vi "Insert Add States to Queue.vi"(8 "error in (no error)":errorcluster, 9 "Mouse Position":T1, 10 "Variant in":path, 11 "?":refnum<vi>) -> (0 "error out":errorcluster)   [LabVIEW 2020]
doc: "Inserts the object specified by name in the Quick Drop dialog box on the selected wire(s) on the diagram. If [Shift] is also pressed, and multiple wires were selected, a single instance of the object is inserted on those wires.\n\nDefault Shortcut - [I]"
uses:
  <vilib>/Utility/miscctls.llb/LVPositionTypeDef.ctl
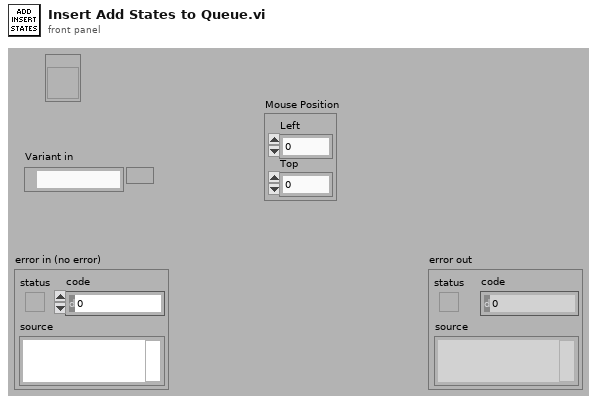
[diagram p1: front panel]
types:
  T1 = typedef "LVPositionTypeDef.ctl" = cluster{"Left":i32, "Top":i32}
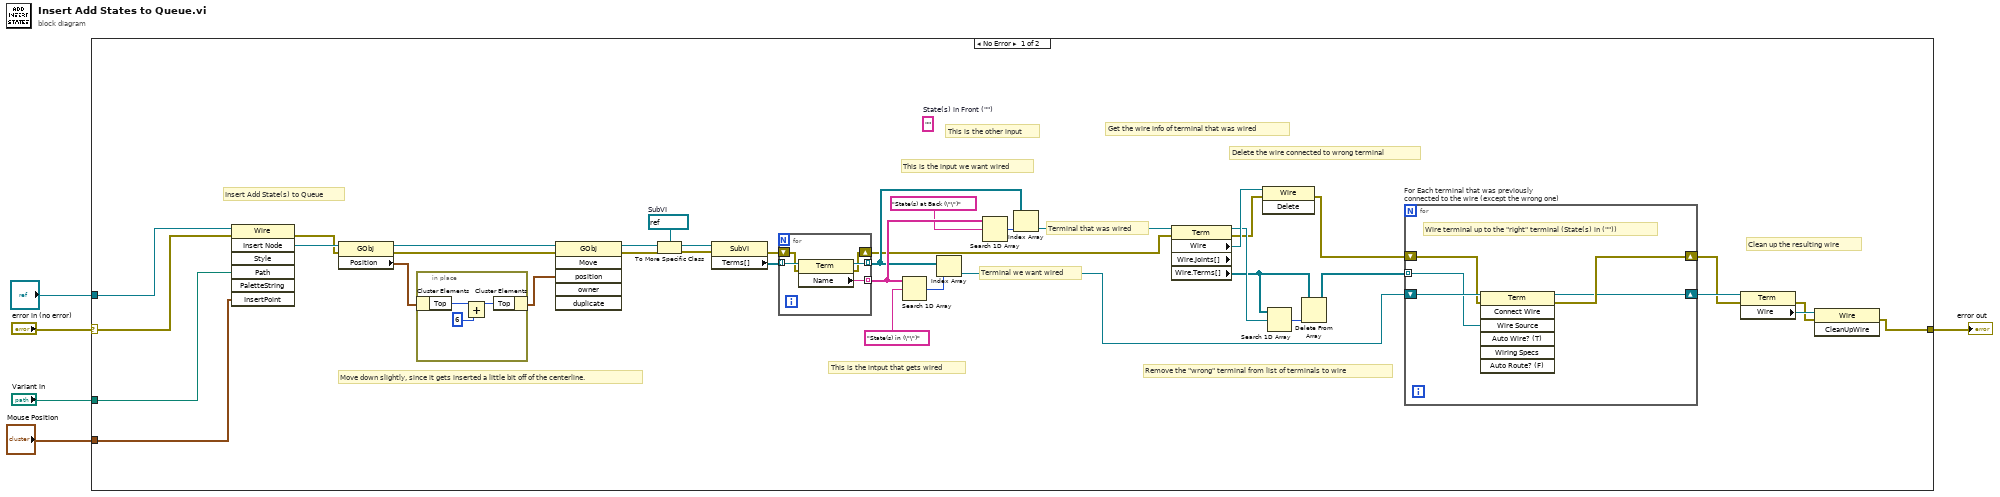
[diagram p0: block diagram]
diagram:
  n1 = case shown="No Error" "error in (no error)" {
    selector: "error in (no error)" -> [w42 w57]
    tunnel: [w43 w57] -> w4
    tunnel: "Variant in" -> [w41 _]
    tunnel: "?" -> [w40 _]
    tunnel: "Mouse Position" -> [w39 _]
    frame No Error {
      w38 = refnum<vi> refnum  # SubVI
      (unwired) ""  # State(s) in Front ("")
      # "Clean up the resulting wire"
      # "Remove the \"wrong\" terminal from list of terminals to wire"
      # "Delete the wire connected to wrong terminal"
      # "Get the wire info of terminal that was wired"
      # "This is the other input"
      # "This is the input we want wired"
      # "This is the intput that gets wired"
      # "Insert Add State(s) to Queue"
      # "Move down slightly, since it gets inserted a little bit off of the centerline."
      # "Terminal that was wired"
      # "Terminal we want wired"
      n2 = invoke class="Wire" method="Insert Node"(reference=w40, error in=w42, "Path"=w41, "InsertPoint"=w39) -> (error out=w11:errorcluster, "Insert Node"=w12:refnum<vi>)  [unwired: 3 in, 5 out]
      n3 = property class="GObj"(reference=w12, error in=w11) -> (reference out=w10:refnum<vi>, error out=w7:errorcluster, "Position"=w13:T1)
      n4 = in-place {
        n5 = in-place-cluster #1(w13) -> ("Top"=w46:i32)
        n6 = Add(x=w46, y=6) -> (x+y=w44:i32)
        n7 = in-place-cluster #1("Top"=w44) -> (w8:T1)
      }
      n8 = invoke class="GObj" method="Move"(reference=w10, error in=w7, "position"=w8) -> (reference out=w9:refnum<vi>, error out=w6:errorcluster)  [unwired: 3 in, 4 out]
      n9 = To More Specific Class(target class=w38, reference=w9, error in=w6) -> (specific class reference=w37:refnum<vi>, error out=w30:errorcluster)
      n10 = property class="SubVI"(reference=w37, error in=w30) -> (error out=w21:errorcluster, "Terms[]"=w36:refnum<vi>[])  [unwired: 1 out]
      n11 = for {
        tunnel: w36 -> [w56] mode=indexing
        tunnel: [w55] -> w34 mode=indexing
        tunnel: [w54] -> w31 mode=indexing
        shift-right: [w52] -> w20
        shift-left: w21 -> [w53]
        n12 = property class="Term"(reference=w56, error in=w53) -> (reference out=w54:refnum<vi>, error out=w52:errorcluster, "Name"=w55:string)
      }
      n13 = Search 1D Array(1D array=w34, element="State(s) in (\"\")") -> (index of element=w28:i32)  [unwired: 1 in]
      n14 = Index Array(array=w31, index=w28) -> (element=w22:refnum<vi>)
      n15 = Search 1D Array(1D array=w34, element="State(s) at Back (\"\")") -> (index of element=w32:i32)  [unwired: 1 in]
      n16 = Index Array(array=w31, index=w32) -> (element=w29:refnum<vi>)
      n17 = property class="Term" props=["Wire", "Wire", "Joints[]", "Wire", "Terms[]"](reference=w29, error in=w20) -> (reference out=w26:refnum<vi>, error out=w19:errorcluster, "Wire"=w27:refnum<vi>, "Wire.Terms[]"=w24:refnum<vi>[])  [unwired: 1 out]
      n18 = invoke class="Wire" method="Delete"(reference=w27, error in=w19) -> (error out=w18:errorcluster)  [unwired: 1 in, 2 out]
      n19 = Search 1D Array(1D array=w24, element=w26) -> (index of element=w25:i32)  [unwired: 1 in]
      n20 = Delete From Array(array=w24, index=w25) -> (array with subset deleted=w23:refnum<vi>[])  [unwired: 1 in, 1 out]
      n21 = for "For Each terminal that was previously connected to the wire (except the wrong one)" {
        tunnel: w23 -> [w50] mode=indexing
        shift-right: [w48] -> w14
        shift-left: w18 -> [w49]
        shift-right: [w47] -> w17
        shift-left: w22 -> [w51]
        # "Wire terminal up to the \"right\" terminal (State(s) in (\"\"))"
        n22 = invoke class="Term" method="Connect Wire"(reference=w51, error in=w49, "Wire Source"=w50) -> (reference out=w47:refnum<vi>, error out=w48:errorcluster)  [unwired: 4 in, 5 out]
      }
      n23 = property class="Term"(reference=w17, error in=w14) -> (error out=w15:errorcluster, "Wire"=w16:refnum<vi>)  [unwired: 1 out]
      n24 = invoke class="Wire" method="CleanUpWire"(reference=w16, error in=w15) -> (error out=w43:errorcluster)  [unwired: 1 in, 2 out]
    }
    frame Error {
    }
  }
  "error out" <- w4
